vi "Tab Delimiter.vi"(8 "Error In":errorcluster) -> (0 "Error Out":errorcluster)   [LabVIEW 2018, in "Tests.lvlib"]
uses:
  Tests.lvlib
  src/Toolkit/Support/Manager.vi
  <vilib>/addons/_JKI Toolkits/Caraya/classes/Test/Test.lvclass
  <vilib>/addons/_JKI Toolkits/Caraya/classes/Assert/Assert.lvclass
  src/Toolkit/Toolkit.lvlib
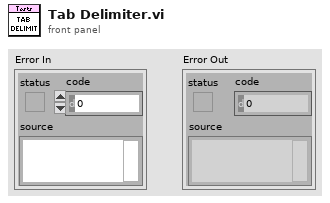
[diagram p1: front panel]
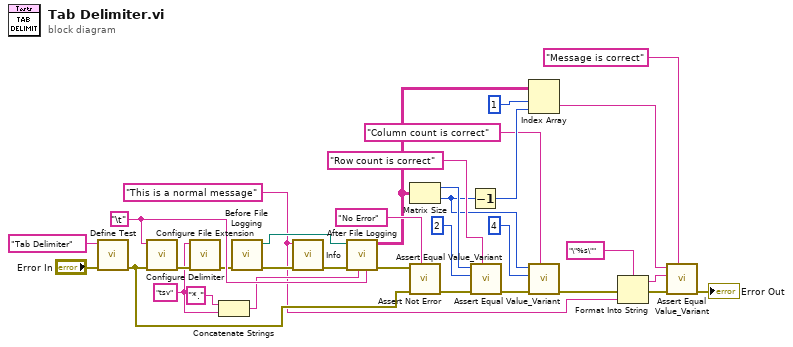
[diagram p0: block diagram]
diagram:
  w11 = "tsv" ("File Extension")
  w15 = "\t"
  w7 = "This is a normal message" ("Message")
  n1 = call <vilib>:"Define Test.vi"("error in (no error)"="Error In", "Label (VI Title)"="Tab Delimiter") -> ("error out"=w32:errorcluster)  [unwired: 9 in]
  n2 = call "Configure Delimiter.vi"("Error In"=w32, "Delimiter"=w15) -> ("Error Out"=w14:errorcluster)  [unwired: 9 in]
  n3 = call "Configure File Extension.vi"("Error In"=w14, "File Extension"=w11) -> ("Error Out"=w13:errorcluster)  [unwired: 9 in]
  n4 = Concatenate Strings("*." ("string"), w11) -> (w10:string)
  n5 = call "Before File Logging.vi"("Error In"=w13) -> ("Error Out"=w30:errorcluster, "Test Log Folder"=w26:path)  [unwired: 9 in]
  n6 = call "Info.vi"("Error In"=w30, "Message"=w7) -> ("Error Out"=w29:errorcluster)  [unwired: 9 in]
  n7 = call "After File Logging.vi"("Delimiter"=w15, "List Folder Pattern"=w10, "Error In"=w29, "Test Log Folder"=w26) -> ("Error Out"=w25:errorcluster, "Records"=w21:string[][])  [unwired: 6 in]
  n8 = Matrix Size(0:w21) -> (1:w24:i32, 2:w3:i32)
  n9 = call <vilib>:"Assert Not Error.vi"("Label"="No Error", "error in (no error)"=w32, "Not Error?"=w25) -> ("error out"=w27:errorcluster)  [unwired: 8 in]
  n10 = Decrement(x=w3) -> (x-1=w19:i32)
  n11 = call <vilib>:"Assert Equal Value_Variant.vi"("Label"="Row count is correct", "error in (no error)"=w27, "Y"=2 ("size(s)"), "X"=w24) -> ("error out"=w5:errorcluster)  [unwired: 7 in]
  n12 = Index Array(array=w21, index (row)=1, index (col)=w19) -> (element=w16:string)
  n13 = call <vilib>:"Assert Equal Value_Variant.vi"("Label"="Column count is correct", "error in (no error)"=w5, "Y"=4 ("number of columns"), "X"=w3) -> ("error out"=w4:errorcluster)  [unwired: 7 in]
  n14 = Format Into String(format string="\"%s\"", error in=w4, w7) -> (resulting string=w6:string, error out=w9:errorcluster)  [unwired: 1 in]
  n15 = call <vilib>:"Assert Equal Value_Variant.vi"("Label"="Message is correct", "error in (no error)"=w9, "Y"=w6, "X"=w16) -> ("error out"=→"Error Out":errorcluster)  [unwired: 7 in]
